vi "DataStream_PC_Build Plot Names.vi"(10 "Name Array Out":string[](array[string]), 11 "XYGraph in":refnum<vi>) -> ()   [LabVIEW 2020]
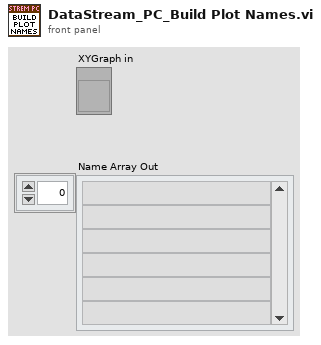
[diagram p1: front panel]
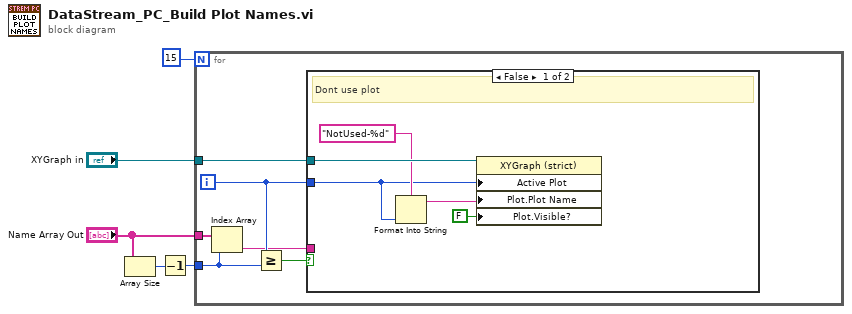
[diagram p0: block diagram]
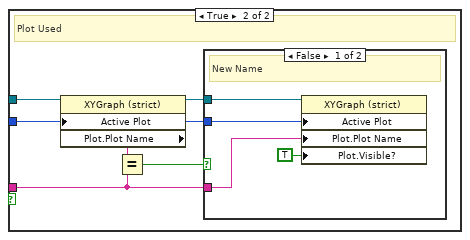
[diagram p2: hidden frame]
diagram:
  n1 = Array Size(array="Name Array Out") -> (size(s)=w3:i32)
  n2 = Decrement(x=w3) -> (x-1=w4:i32)
  n3 = for {
    N: 15 -> [_]
    tunnel: "Name Array Out" -> [w11]
    tunnel: w4 -> [w8]
    tunnel: "XYGraph in" -> [w10]
    i -> [w9]
    n4 = Index Array(array=w11, index=w8) -> (element=w6:string)
    n5 = Greater Or Equal?(x=w9, y=w8) -> (x >= y?=w7:bool)
    n6 = case shown="False" w7 {
      tunnel: w10 -> [w16 w22]
      tunnel: w9 -> [w14 w18]
      tunnel: w6 -> [_ w17]
      frame False {
        # "Dont use plot"
        n7 = Format Into String(format string="NotUsed-%d", w14) -> (resulting string=w13:string)  [unwired: 2 in, 1 out]
        n8 = property on="Property Node" class="XYGraph (strict)"(reference=w16, "Active Plot"=w14, "Plot.Plot Name"=w13, "Plot.Visible?"=FALSE ("Plot.Visible")) -> ()  [unwired: 1 in, 2 out]
      }
      frame True {
        # "Plot Used"
        n9 = property on="Property Node" class="XYGraph (strict)"(reference=w22, "Active Plot"=w18) -> (reference out=w19:refnum<vi>, "Plot.Plot Name"=w21:string)  [unwired: 1 in, 1 out]
        n10 = Equal?(x=w21, y=w17) -> (x = y?=w20:bool)
        n11 = case shown="False" w20 {
          tunnel: w19 -> [w26 _]
          tunnel: w18 -> [w25 _]
          tunnel: w17 -> [w24 _]
          frame False {
            # "New Name"
            n12 = property on="Property Node" class="XYGraph (strict)"(reference=w26, "Active Plot"=w25, "Plot.Plot Name"=w24, "Plot.Visible?"=TRUE ("Plot.Visible")) -> ()  [unwired: 1 in, 2 out]
          }
          frame True {
            # "Same Name"
          }
        }
      }
    }
  }
